vi "Get Tree.vi"(8 "error in (no error)":errorcluster, 11 "PathTreeNode in":refnum<class "PathTreeNode.lvclass">) -> (0 "error out":errorcluster, 2 "Tree":refnum<class "PathTree.lvclass">, 3 "PathTreeNode out":refnum<class "PathTreeNode.lvclass">)   [LabVIEW 2020, in "PathTree.lvlib" / "PathTreeNode.lvclass"]
uses:
  PathTreeNode.lvclass
  PathTree/PathTree.lvclass
  PathTreeNode.lvclass/PathTreeNode.ctl
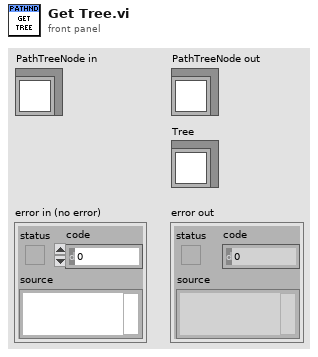
[diagram p1: front panel]
types:
  T1 = typedef "Advanced Structures.lvlib/PathTreeNode.lvclass/Ref Data.ctl" = cluster{"Tree":refnum<class>, "Parent":refnum<class>, "Token":string, "Child Tokens":string[], "Child Nodes":refnum<class>[], "Value":refnum<class>, "Has Value":bool}
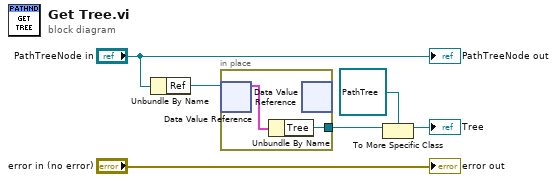
[diagram p0: block diagram]
diagram:
  n1 = Unbundle By Name("PathTreeNode in") -> ("Ref"=w5:refnum<data-value>)
  n2 = in-place {
    in-place-border: [w7] -> w3
    n3 = in-place-dvr #1(w5) -> (w8:T1)  [unwired: 1 out]
    n4 = Unbundle By Name(w8) -> ("Tree"=w7:refnum<class>)
    n5 = in-place-dvr #1() -> ()  [unwired: 1 in, 2 out]
  }
  n6 = To More Specific Class(target class=refnum<class "PathTree.lvclass"> refnum ("Advanced Structures.lvlib:PathTree.lvclass"), reference=w3) -> (specific class reference=→"Tree":refnum<class "PathTree.lvclass">)  [unwired: 1 in, 1 out]
  "error out" <- "error in (no error)"
  "PathTreeNode out" <- "PathTreeNode in"
